vi "Enable State Auto Recall.vi"(8 "error in (no error)":errorcluster, 10 "Enable Auto Recall (T: Enable)":bool=TRUE, 11 "VISA resource name":refnum<visa-resource-name>) -> (0 "error out":errorcluster, 3 "VISA resource name out":refnum<visa-resource-name>)   [LabVIEW 2010, in "AWG.lvlib" / "Agilent 3352X Series.lvlib"]
doc: "Disables or enables the automatic recall of a specific stored instrument state from storage location \"0\" when power is turned on."
uses:
  Agilent 3352X Series.lvlib
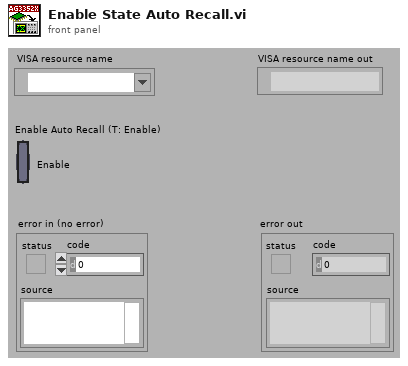
[diagram p1: front panel]
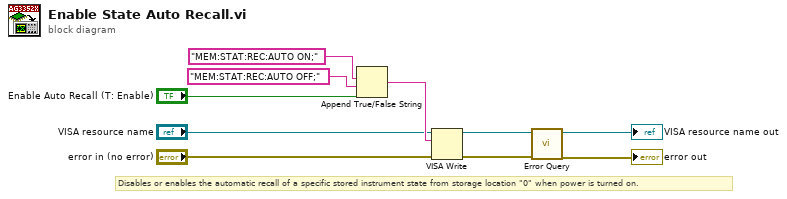
[diagram p0: block diagram]
diagram:
  # "Disables or enables the automatic recall of a specific stored instrument state from storage location \"0\" when power is turned on."
  n1 = Append True/False String(1:"Enable Auto Recall (T: Enable)", 2:"MEM:STAT:REC:AUTO OFF;", 3:"MEM:STAT:REC:AUTO ON;") -> (0:w7:string)  [unwired: 1 out]
  n2 = VISA Write(VISA resource name="VISA resource name", write buffer=w7, error in (no error)="error in (no error)") -> (VISA resource name out=w4:refnum<visa-resource-name>, error out=w3:errorcluster)  [unwired: 1 out]
  n3 = call "Error Query.vi"("error in (no error)"=w3, "VISA resource name"=w4) -> ("error out"=→"error out":errorcluster, "VISA resource name out"=→"VISA resource name out":refnum<visa-resource-name>)  [unwired: 8 out]
